vi "Set Control Custom Symbols with Index File (Tree)__Uti.vi"(8 "error in (no error)":errorcluster, 10 "custom symbol files with indice":cluster{"Index":i32, "Picture Path":path}[](array[cluster]), 11 "tree in":refnum<vi>) -> (0 "error out":errorcluster, 3 "tree out":refnum<vi>)   [LabVIEW 2012]
doc: "用Index和图片文件路径组成的簇设置树控件的Custom Symbol。图片文件所接受的格式包括jpeg、bmp、png"
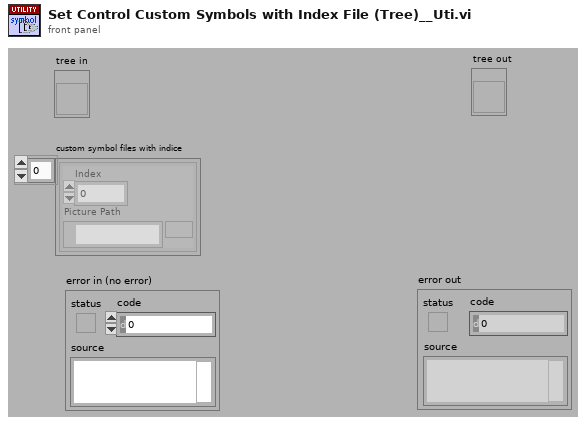
[diagram p1: front panel]
types:
  T1 = typedef "imagedata.ctl" = cluster{"image type":i32, "image depth":i32, "image":u8[], "mask":u8[], "colors":u32[], "Rectangle":cluster{"left":i16, "top":i16, "right":i16, "bottom":i16}}
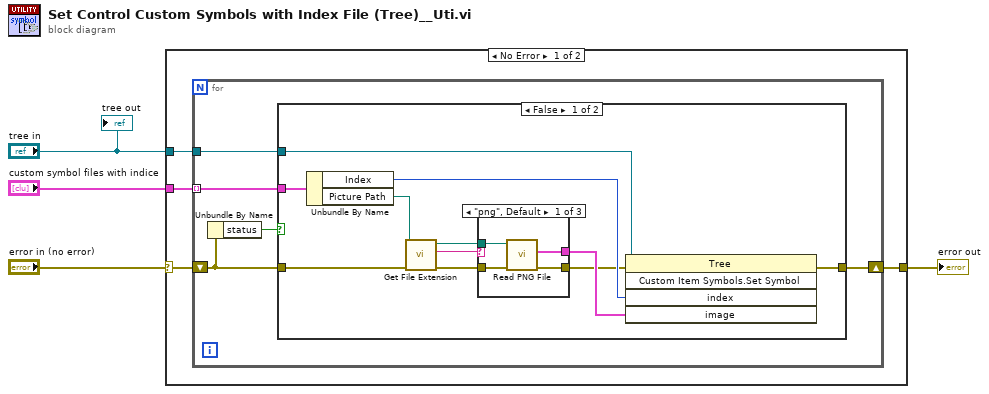
[diagram p0: block diagram]
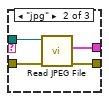
[diagram p2: hidden frame]
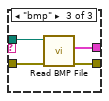
[diagram p3: hidden frame]
diagram:
  n1 = case shown="No Error" "error in (no error)" {
    selector: "error in (no error)" -> [w6 w38]
    tunnel: "tree in" -> [w8 _]
    tunnel: "custom symbol files with indice" -> [w7 _]
    tunnel: [w5 w38] -> w1
    frame No Error {
      n2 = for {
        tunnel: w8 -> [w13]
        tunnel: w7 -> [w12] mode=indexing
        shift-right: [w9] -> w5
        shift-left: w6 -> [w10]
        n3 = Unbundle By Name(w10) -> ("status"=w11:bool)
        n4 = case shown="False" w11 {
          tunnel: w13 -> [w24 _]
          tunnel: w12 -> [w23 _]
          tunnel: w10 -> [w20 w37]
          tunnel: [w14 w37] -> w9
          frame False {
            n5 = Unbundle By Name(w23) -> ("Index"=w21:i32, "Picture Path"=w22:path)
            n6 = call <vilib>:"Get File Extension.vi"("error in (no error)"=w20, "file"=w22) -> ("error out"=w17:errorcluster, "lowercase file extension"=w19:string, "dup file"=w18:path)  [unwired: 7 out]
            n7 = case shown="\"png\", Default" w19 {
              tunnel: w18 -> [w28 w32 w36]
              tunnel: w17 -> [w27 w31 w35]
              tunnel: [w26 w30 w33] -> w16
              tunnel: [w25 w29 w34] -> w15
              frame "png", Default {
                n8 = call <vilib>:"Read PNG File.vi"("error in (no error)"=w27, "path to PNG file"=w28) -> ("error out"=w25:errorcluster, "image data"=w26:T1)  [unwired: 8 out]
              }
              frame "jpg" {
                n9 = call <vilib>:"Read JPEG File.vi"("error in (no error)"=w31, "path to JPEG file"=w32) -> ("error out"=w29:errorcluster, "image data"=w30:T1)  [unwired: 8 out]
              }
              frame "bmp" {
                n10 = call <vilib>:"Read BMP File.vi"("error in (no error)"=w35, "path to BMP file"=w36) -> ("error out"=w34:errorcluster, "image data"=w33:T1)  [unwired: 8 out]
              }
            }
            n11 = invoke on="Invoke Node" class="Tree" method="Custom Item Symbols.Set Symbol"(reference=w24, error in=w15, "index"=w21, "image"=w16) -> (error out=w14:errorcluster)  [unwired: 1 in, 4 out]
          }
          frame True {
          }
        }
      }
    }
    frame Error {
    }
  }
  "error out" <- w1
  "tree out" <- "tree in"
